vi "Append Value To Waveform.vi"(10 "Numeric":dbl, 11 "waveform in":waveform(dbl)) -> (3 "waveform out":waveform(dbl))   [LabVIEW 2017, in "Logger.lvclass"]
uses:
  logger/Logger.lvclass
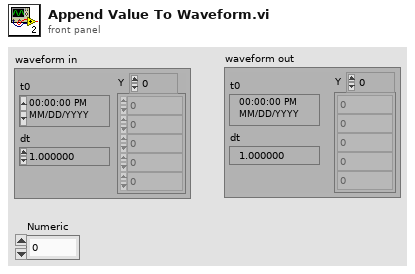
[diagram p1: front panel]
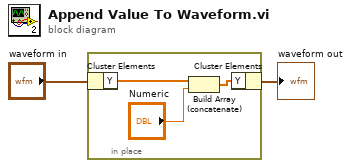
[diagram p0: block diagram]
diagram:
  n1 = in-place {
    n2 = in-place-cluster #1("waveform in") -> ("Y"=w4:dbl[])
    n3 = Build Array (concatenate)(w4, "Numeric") -> (w3:dbl[])
    n4 = in-place-cluster #1("Y"=w3) -> (→"waveform out":waveform(dbl))
  }
